vi "Get Date.vi"(7 "Optional":bool, 8 "error in (no error)":errorcluster, 9 "Default":timestamp, 10 "Name":string, 11 "LV Argument Parser in":refnum<class "LV Argument Parser.lvclass">) -> (0 "error out":errorcluster, 1 "Value":timestamp, 2 "key not found?":bool, 3 "LV Argument Parser out":refnum<class "LV Argument Parser.lvclass">)   [LabVIEW 2020, in "LV ArgParse.lvlib" / "LV Argument Parser.lvclass"]
uses:
  LV Argument Parser.lvclass
  LV Argument Parser.lvclass/LV Argument Parser.ctl
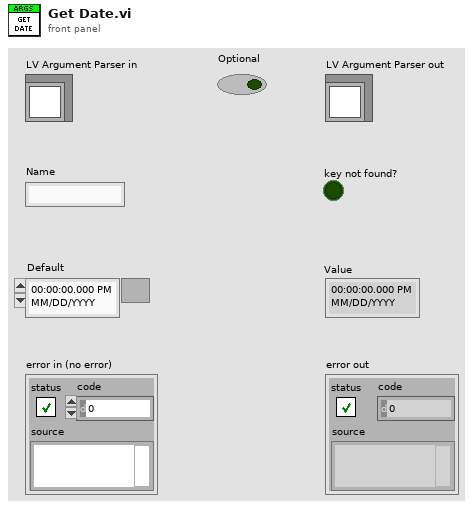
[diagram p1: front panel]
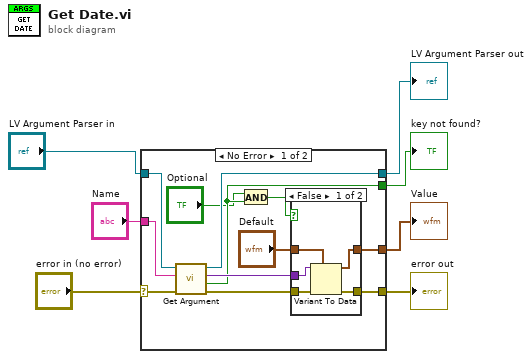
[diagram p0: block diagram]
diagram:
  n1 = case shown="No Error" "error in (no error)" {
    selector: "error in (no error)" -> [w19 w28]
    tunnel: [w14 w28] -> w6
    tunnel: [w16 w27] -> w4
    tunnel: "LV Argument Parser in" -> [w17 w27]
    tunnel: "Name" -> [w15 _]
    tunnel: [w11 _] -> w2
    tunnel: [w12 _] -> w1
    frame No Error {
      n2 = call "Get Argument.vi"("error in (no error)"=w19, "Name"=w15, "LV Argument Parser in"=w17) -> ("error out"=w18:errorcluster, "key not found?"=w11:bool, "element"=w13:variant, "LV Argument Parser out"=w16:refnum<class "LV Argument Parser.lvclass">)  [unwired: 5 in]
      n3 = And(x="Optional", y=w11) -> (x .and. y?=w10:bool)
      n4 = case shown="False" w10 {
        tunnel: w18 -> [w24 w26]
        tunnel: [w23 w26] -> w14
        tunnel: w13 -> [w22 _]
        tunnel: [w21 w25] -> w12
        tunnel: "Default" -> [w20 w25]
        frame False {
          n5 = Variant To Data(error in=w24, type=w20, Variant=w22) -> (data=w21:timestamp, error out=w23:errorcluster)
        }
        frame True {
        }
      }
    }
    frame Error {
    }
  }
  "error out" <- w6
  "LV Argument Parser out" <- w4
  "key not found?" <- w2
  "Value" <- w1
